vi "Param.vi"() -> ()   [LabVIEW 2017]
uses:
  Settings/Traverse-Settings-Global.vi
panel:
  out "mm/rotation":dbl[](array[numeric])
  out "Speed":dbl(knob) scale=0.0..250.0
  out "Degre Factor":dbl[](array[numeric])
  out "Pulse/Degree":dbl
  out "Max Velocity":dbl[](array[numeric])
  out "Deceleration":dbl[](array[numeric])
  out "Acceleration":dbl[](array[numeric])
  in  "stop":bool
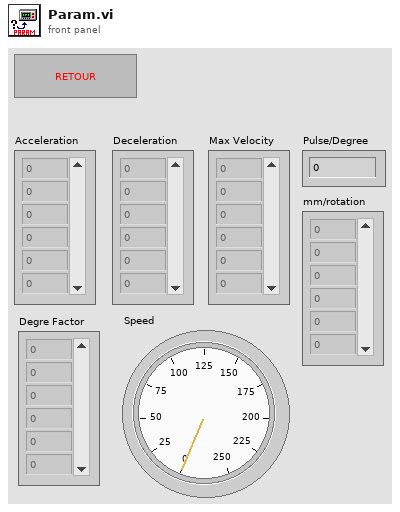
[diagram p1: front panel]
types:
  T1 = typedef "Settings-Control.ctl" = cluster{"Acceleration":dbl[], "Deceleration":dbl[], "Max Velocity":dbl[], "Speed":dbl, "Pulse/Degree":dbl, "Degre Factor":dbl[], "mm/rotation":dbl[], "Traverse Name":string}
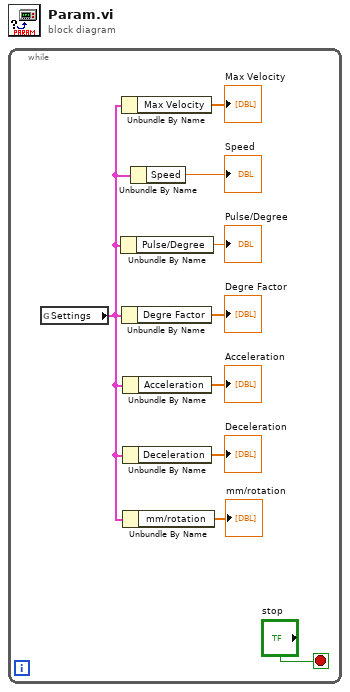
[diagram p0: block diagram]
diagram:
  n1 = while {
    stop <- "stop" stop-if-true
    n2 = global read "Traverse-Settings-Global.vi" "Settings"() -> (w1:T1)
    n3 = Unbundle By Name(w1) -> ("Pulse/Degree"=→"Pulse/Degree":dbl)
    n4 = Unbundle By Name(w1) -> ("Max Velocity"=→"Max Velocity":dbl[])
    n5 = Unbundle By Name(w1) -> ("Degre Factor"=→"Degre Factor":dbl[])
    n6 = Unbundle By Name(w1) -> ("Acceleration"=→"Acceleration":dbl[])
    n7 = Unbundle By Name(w1) -> ("Deceleration"=→"Deceleration":dbl[])
    n8 = Unbundle By Name(w1) -> ("mm/rotation"=→"mm/rotation":dbl[])
    n9 = Unbundle By Name(w1) -> ("Speed"=→"Speed":dbl)
  }
